vi "add subvi.vi"(1 "b":dbl, 2 "a":dbl) -> (0 "x+y":dbl)   [LabVIEW 2025]
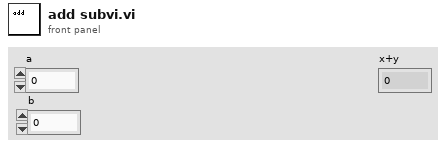
[diagram p1: front panel]
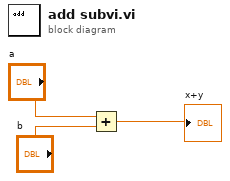
[diagram p0: block diagram]
diagram:
  n1 = Add(x="a", y="b") -> (x+y=→"x+y":dbl)
